vi "generate user events.vi"(8 "error in (no error)":errorcluster, 11 "Template in":refnum<class "Template.lvclass">) -> (0 "error out":errorcluster, 3 "Template out":refnum<class "Template.lvclass">)   [LabVIEW 2020, in "Template.lvlib" / "Template.lvclass"]
uses:
  Template.lvclass
  typedefs/base actor events.ctl
  Template.lvclass/Template.ctl
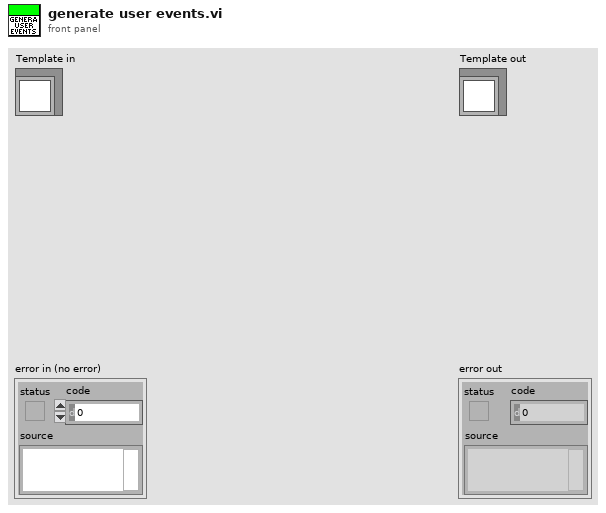
[diagram p1: front panel]
types:
  T1 = typedef "Template.lvlib/Template.lvclass/base actor events.ctl" = cluster{"Stop Actor":refnum<user-event>, "New Error":refnum<user-event>}
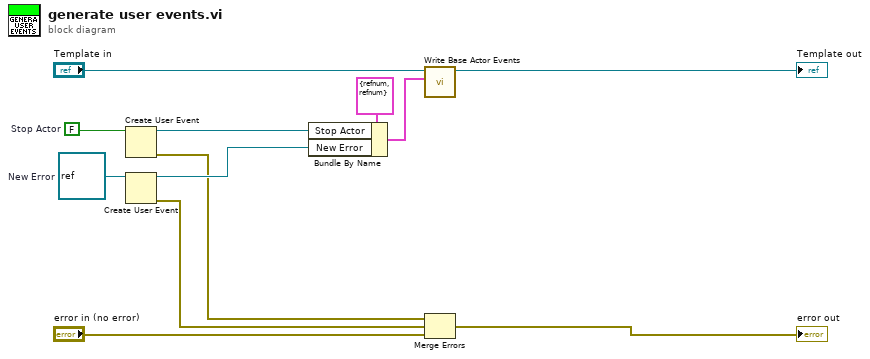
[diagram p0: block diagram]
diagram:
  w5 = refnum<class> refnum  # New Error
  w10 = FALSE  # Stop Actor
  n1 = Create User Event(user event datatype=w10) -> (user event=w6:refnum<user-event>, error out=w1:errorcluster)  [unwired: 1 in]
  n2 = Create User Event(user event datatype=w5) -> (user event=w4:refnum<user-event>, error out=w2:errorcluster)  [unwired: 1 in]
  n3 = Bundle By Name(cluster=T1 {"Stop Actor"=refnum, "New Error"=refnum} ("Base Actor Events"), "Stop Actor"=w6, "New Error"=w4) -> (w7:T1)
  n4 = call "Write Base Actor Events.vi"("Base Actor Events"=w7, "Template in"="Template in") -> ("Template out"=→"Template out":refnum<class "Template.lvclass">)  [unwired: 9 in]
  n5 = Merge Errors(w1, w2, "error in (no error)") -> (→"error out":errorcluster)
